vi "Drivetrain Loop.vi"   [LabVIEW 2016]
uses:
  <vilib>/Rock Robotics/WPI/ThirdParty/Sensors/navX/_TypeDefs/FRIC_navX_DeviceNumbersTypeDef.ctl
  Common Code/PID Gains.ctl
  Common Code/Utilities/Change Detect Int.vi
  Common Code/Utilities/Change Detect Boolean.vi
  Robot Global Data.vi
  <vilib>/Rock Robotics/WPI/Solenoid/Deprecated/WPI_SolenoidSetBool.vi
types:
  T1 = typedef "FRIC_navX_DeviceNumbersTypeDef.ctl" = enum16{"Dev0", "Dev1", "Dev2", "Dev3"}
  T2 = typedef "Drivetrain Command Cluster.ctl" = cluster{"Drivetrain Mode":T3, "Heading Target":dbl, "Turn Power":dbl, "Y Power":dbl, "Center Piston Down?":bool, "Traction?":bool, "Strafe Power":dbl, "Zero Gyro":bool, "Distance Target":dbl, "Strafe Correct":bool, "Y Max Output":dbl, "Y Min Output":dbl, "X Max Output":dbl, "X Min Output":dbl, "Z Max Output":dbl, "Z Min Output":dbl, "Z Target":dbl, "Brake?":bool}
  T3 = typedef "Drivetrain Mode.ctl" = enum16{"Manual", "Gyro Steer", "Distance Drive", "Translate Drive", "Goal Vision Align", "PID Drive"}
  T4 = typedef "Dashboard Control Data.ctl" = cluster{"Drivetrain Settings":T5, "Intake Presets ":T8, "Shooter Presets":T9, "Vision Target Packet":T10, "Auton Presets":cluster{"Start Position":dbl}, "Drivetrain Encoder Values":T11, "Drivetrain Encoder Settings":cluster{"Left Tick Constant":dbl, "Right Tick Contant":dbl, "Reset Encoders":bool, "Center Tick Constant":dbl}, "Zero Gyro":bool, "Vision Timeout":dbl, "Pressure M":dbl, "Pressure B":dbl, "Auto Agitator":T13, "Climber Settings":T14, "LEDs":T15}
  T5 = typedef "Drivetrain Settings.ctl" = cluster{"Gyro Tolerance":dbl, "Gyro Steer PID Gains":T6, "Y Power Multiplier":dbl, "Turn Power Multiplier":dbl, "Gyro Output":dbl, "Creep Rate":dbl, "Distance Drive PID Gains":T6, "Distance Tolerance":dbl, "Distance Output":dbl, "Strafe Threshold":dbl, "Strafe Correct":bool, "Strafe Corect Tolerance":dbl, "Translate Drive PID Gains":T6, "Strafe Output":dbl, "SC Right":dbl, "SC Left":dbl, "Use Gyro":bool, "Constant Power":bool, "Strafe Power":dbl, "Input Modifier":T7}
  T6 = typedef "PID Gains.ctl" = cluster{"proportional gain (Kc)":dbl, "integral time (Ti, min)":dbl, "derivative time (Td, min)":dbl}
  T7 = typedef "Input Modifier.ctl" = enum16{"None", "Square", "Cube"}
  T8 = typedef "Intake Presets.ctl" = cluster{"Intake Speed ":dbl, "Outake Speed":dbl, "Current Trip Delay":dbl, "Max Current":dbl, "Gear Outtake Motor Delay":dbl, "Gear Intake Motor Delay":dbl, "Gear Intake?":bool, "Gear Intake Pull Up Speed":dbl}
  T9 = typedef "Shooter Presets.ctl" = cluster{"Key Shot":cluster{"RPM ":dbl, "Hood?":bool}, "Distance Shot":cluster{"RPM":dbl, "Hood?":bool}, "RPM Tolerance":dbl, "Unstuck Delay Time ":dbl, "Initial RPM Increase":dbl, "Warmup Delay":dbl, "Faster Time":dbl, "Shooter PID Gains":cluster{"P":dbl, "I":dbl, "D":dbl, "FF":dbl, "Ramp Rate":dbl, "I Zone":dbl}, "Unstuck Trigger Power":dbl, "Trigger Power":dbl, "Unstuck RPM":dbl, "Agitator Active Power":dbl, "Agitator Idle Power":dbl}
  T10 = typedef "Vision Target Packet.ctl" = cluster{"Robot Center":dbl, "Center X":dbl, "Center Y":dbl, "Angle":dbl, "Distance":dbl, "Found Target?":bool}
  T11 = typedef "Drivetrain Encoder Values.ctl" = cluster{"Left Encoder":T12, "Center Encoder":T12, "Right Encoder":T12}
  T12 = typedef "Encoder Values.ctl" = cluster{"Distance":dbl, "Speed":dbl, "Tick":dbl}
  T13 = typedef "Auto Agitator Settings.ctl" = cluster{"Enable Auto Agitation":bool, "Continuous Stir":bool, "Continuous Intake":bool, "Alternate In/Outtake":bool, "Wing Delay":dbl, "Stir Delay":dbl, "Intake Delay":dbl, "Wing On Time":dbl, "Wing Off Time":dbl, "Stir On Time":dbl, "Stir Off Time":dbl, "Intake On Time":dbl, "Intake Off Time":dbl, "Stir Power":dbl, "Intake Power":dbl, "Outtake Power":dbl, "Intake Run Time":dbl, "Outtake Run Time":dbl, "Wing$":bool, "Intake":bool, "Stirrer":bool}
  T14 = typedef "Climber Settings.ctl" = cluster{"Climber Power":dbl, "Max Current":dbl, "Avoid Current Trip?":bool}
  T15 = typedef "LED Global Data.ctl" = cluster{"Back":cluster{"Default":string, "Traction":string, "Gear Ready":string, "Break On":string, "Gear Loaded":string}, "Front":cluster{"Default":string, "Traction":string, "Gear Ready":string, "Break On":string, "Gear Loaded":string}}
  T16 = typedef "Goal Vision Packet.ctl" = cluster{"Distance":dbl, "Angle":dbl, "Found Target?":bool}
  T17 = cluster{"Yaw":dbl, "Roll":dbl, "Pitch":dbl, "Heading":dbl, "Fused Heading":dbl}
  T18 = cluster{"Target Heading":dbl, "Target Distance":dbl, "Target Translation":dbl}
  T19 = cluster{"Gyro PID Gains":T6, "Distance PID Gains":T6, "Strafe PID Gains":T6}
  T20 = cluster{"Y Max":dbl, "X Max":dbl, "Z Max":dbl, "Y Min":dbl, "X Min":dbl, "Z Min":dbl}
  T21 = cluster{"Distance Tolerance":dbl, "Strafe Tolerance":dbl, "Gyro Tolerance":dbl}
  T22 = typedef "WPI_SolenoidDevRef.ctl" = cluster{"DevStatus":errorcluster, "Pneumatics Control Module":u8, "Forward Solenoid Channel":T23, "Reverse Solenoid Channel":T23}
  T23 = typedef "WPI_SolenoidChannel.ctl" = enum8{"Solenoid 0", "Solenoid 1", "Solenoid 2", "Solenoid 3", "Solenoid 4", "Solenoid 5", "Solenoid 6", "Solenoid 7", "Invalid"}
  T24 = typedef "WPI_MotorControlDeviceRef.ctl" = cluster{"DeviceStatus":errorcluster, "Type":T25, "PWM":cluster{"PWM Channel":T26, "DeadBand":T27}, "CAN":cluster{"Device Number":u8, "SetOutput VI Ref":variant, "GetOutput VI Ref":variant, "Enable VI Ref":variant, "Disable VI Ref":variant, "Data":variant}, "Invert":bool}
  T25 = typedef "WPI_MotorControlType.ctl" = enum16{"PWM", "CAN"}
  T26 = typedef "FPGA_DIOPWMChannel.ctl" = enum8{"PWM 0", "PWM 1", "PWM 2", "PWM 3", "PWM 4", "PWM 5", "PWM 6", "PWM 7", "PWM 8", "PWM 9", "PWM MXP 0", "PWM MXP 1", "PWM MXP 2", "PWM MXP 3", "PWM MXP 4", "PWM MXP 5", "PWM MXP 6", "PWM MXP 7", "PWM MXP 8", "PWM MXP 9", "Invalid"}
  T27 = typedef "WPI_PWMDeadband.ctl" = cluster{"Name":string, "maxPositivePwm":i32, "minPositivePwm":i32, "centerPwm":i32, "maxNegativePwm":i32, "minNegativePwm":i32, "angularRange":u16}
  T28 = typedef "Drivetrain Status Cluster.ctl" = cluster{"Drivetrain Mode":enum16{"Manual", "Gyro Steer"}, "Y (Throttle)":dbl, "X (Steer)":dbl, "Z (Strafe)":dbl, "Heading Target":dbl, "Center Piston Down?":bool, "Traction?":bool, "Gyro Steer Finished?":bool, "Distance Drive Finished?":bool, "Gyro":dbl, "Distance Target":dbl, "Y Max Output":dbl, "Y Min Output":dbl, "X Max Output":dbl, "X Min Output":dbl, "Z Max Output":dbl, "Z Min Output":dbl, "Translation Target":dbl, "Translation Drive Finished?":bool, "PID Auto Drive Finished?":bool, "Brake?":bool, "Vision Aligned?":bool, "Creep Mode Engaged?":bool}
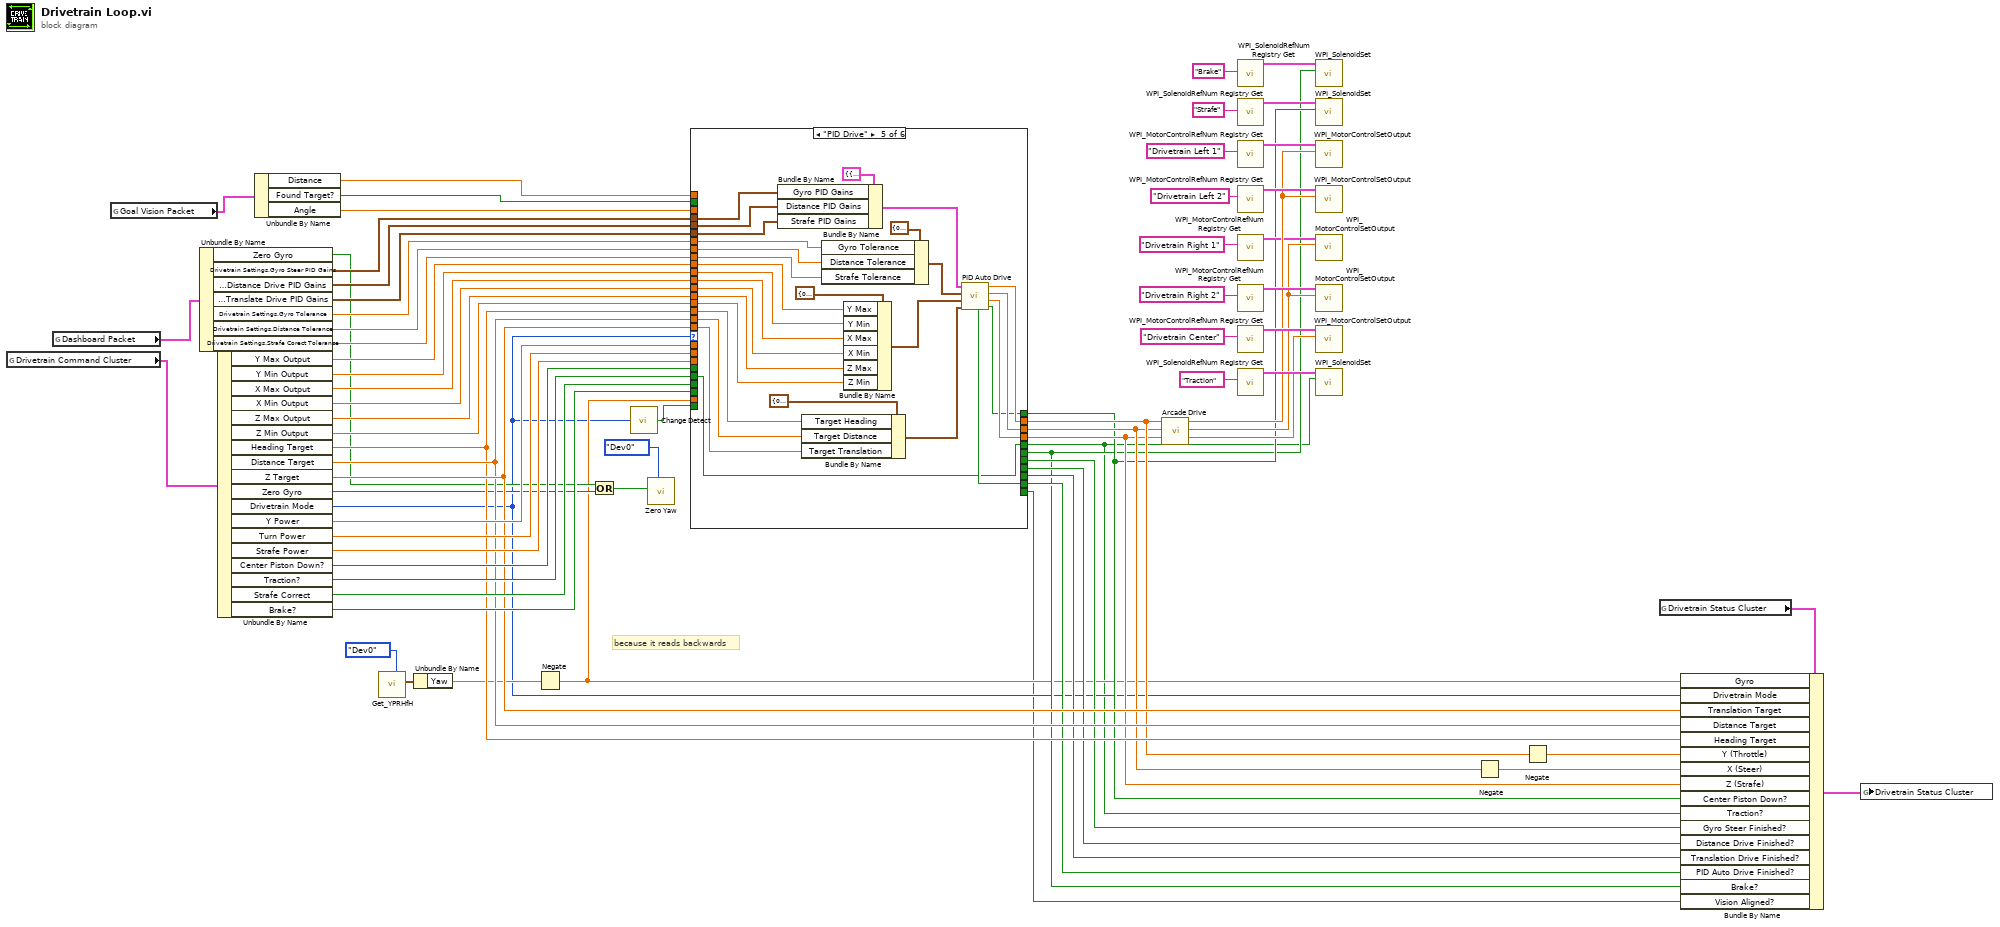
[diagram p0: block diagram]
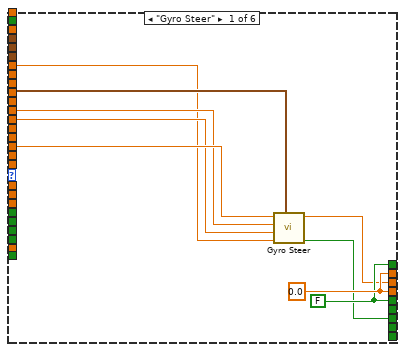
[diagram p2: hidden frame]
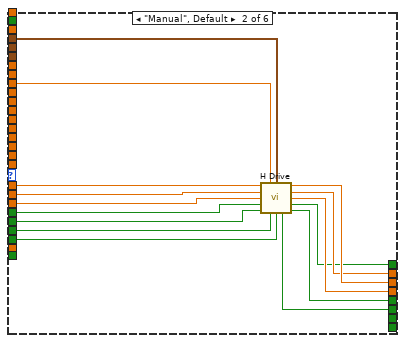
[diagram p3: hidden frame]
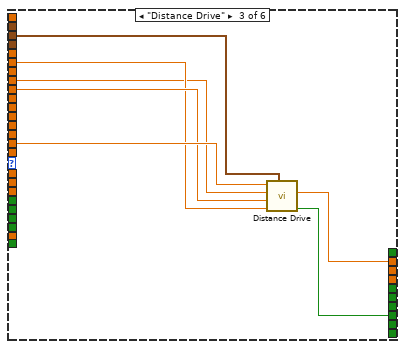
[diagram p4: hidden frame]
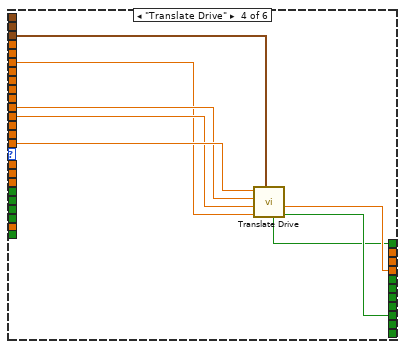
[diagram p5: hidden frame]
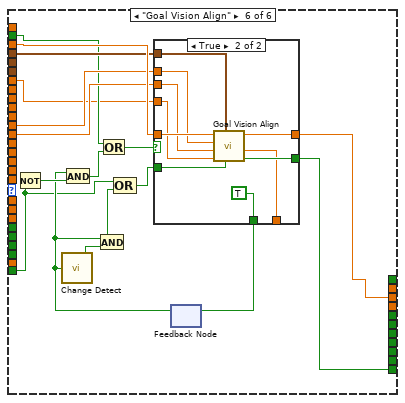
[diagram p6: hidden frame]
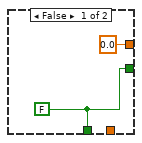
[diagram p7: hidden frame]
diagram:
  # "because it reads backwards"
  n1 = global read "Robot Global Data.vi" "Drivetrain Command Cluster"() -> (w67:T2)
  n2 = global read "Robot Global Data.vi" "Dashboard Packet"() -> (w55:T4)
  n3 = global read "Robot Global Data.vi" "Goal Vision Packet"() -> (w10:T16)
  n4 = Unbundle By Name(w55) -> ("Zero Gyro"=w16:bool, "Drivetrain Settings.Gyro Steer PID Gains"=w54:T6, "Drivetrain Settings.Distance Drive PID Gains"=w53:T6, "Drivetrain Settings.Translate Drive PID Gains"=w42:T6, "Drivetrain Settings.Gyro Tolerance"=w52:dbl, "Drivetrain Settings.Distance Tolerance"=w51:dbl, "Drivetrain Settings.Strafe Corect Tolerance"=w50:dbl)
  n5 = Unbundle By Name(w67) -> ("Y Max Output"=w48:dbl, "Y Min Output"=w47:dbl, "X Max Output"=w45:dbl, "X Min Output"=w46:dbl, "Z Max Output"=w44:dbl, "Z Min Output"=w43:dbl, "Heading Target"=w28:dbl, "Distance Target"=w29:dbl, "Z Target"=w30:dbl, "Zero Gyro"=w17:bool, "Drivetrain Mode"=w4:T3, "Y Power"=w58:dbl, "Turn Power"=w57:dbl, "Strafe Power"=w56:dbl, "Center Piston Down?"=w60:bool, "Traction?"=w59:bool, "Strafe Correct"=w49:bool, "Brake?"=w33:bool)
  n6 = Unbundle By Name(w10) -> ("Distance"=w6:dbl, "Found Target?"=w5:bool, "Angle"=w9:dbl)
  n7 = call <vilib>:"Get_YPRHfH.vi"("Device Number"=FRIC_navX_DeviceNumbersTypeDef."Dev0") -> ("YRPHfH"=w20:T17)  [unwired: 10 in]
  n8 = Unbundle By Name(w20) -> ("Yaw"=w8:dbl)
  n9 = Negate(x=w8) -> (-x=w7:dbl)
  n10 = Or(x=w16, y=w17) -> (x .or. y?=w15:bool)
  n11 = call-poly "Change Detect.vi"("In"=w4) -> ("Changed?"=w3:bool)
  n12 = call <vilib>:"Zero Yaw.vi"("Device Number"=FRIC_navX_DeviceNumbersTypeDef."Dev0", "Zero"=w15) -> ()  [unwired: 10 in]
  n13 = case shown="\"PID Drive\"" w4 {
    tunnel: [w80 w86 w102 _ w115 _] -> w27
    tunnel: [w78 w87 _ _ w114 w140] -> w26
    tunnel: [w80 w85 _ w105 w116 _] -> w25
    tunnel: [w79 w83 _ w103 w113 _] -> w24
    tunnel: [w79 w84 _ _ w111 _] -> w1
    tunnel: w58 -> [_ w95 _ _ _ _]
    tunnel: w57 -> [_ w94 _ _ _ _]
    tunnel: w56 -> [_ w93 _ _ _ _]
    tunnel: w60 -> [_ w92 _ _ _ _]
    tunnel: w59 -> [_ w91 _ _ w111 _]
    tunnel: w54 -> [w76 w90 _ _ w135 w149]
    tunnel: w53 -> [_ _ w100 _ w134 _]
    tunnel: w52 -> [w72 _ _ _ w128 w145]
    tunnel: w51 -> [_ _ w97 _ w127 _]
    tunnel: w28 -> [w75 _ _ _ w119 _]
    tunnel: w29 -> [_ _ w99 _ w118 _]
    tunnel: [w77 _ _ _ _ _] -> w23
    tunnel: [_ _ w101 _ _ _] -> w22
    tunnel: w50 -> [_ w89 _ w106 w126 _]
    tunnel: w49 -> [_ w88 _ _ _ _]
    tunnel: w48 -> [_ _ w96 _ w125 _]
    tunnel: w47 -> [_ _ w98 _ w124 _]
    tunnel: w45 -> [w74 _ _ _ w123 w148]
    tunnel: w46 -> [w73 _ _ _ w122 w147]
    tunnel: w44 -> [_ _ _ w108 w121 _]
    tunnel: w43 -> [_ _ _ w107 w120 _]
    tunnel: w42 -> [_ _ _ w110 w133 _]
    tunnel: w30 -> [_ _ _ w109 w117 _]
    tunnel: [_ _ _ w104 _ _] -> w21
    tunnel: w33 -> [_ w82 _ _ _ _]
    tunnel: [_ w81 _ _ _ _] -> w11
    tunnel: [_ _ _ _ w112 _] -> w12
    tunnel: w9 -> [_ _ _ _ _ w156]
    tunnel: w7 -> [_ _ _ _ _ _]
    tunnel: w6 -> [_ _ _ _ _ _]
    tunnel: w5 -> [_ _ _ _ _ w146]
    tunnel: w3 -> [_ _ _ _ _ w143]
    tunnel: [_ _ _ _ _ w141] -> w2
    frame "Gyro Steer" {
      w80 = 0.0 ("Center Motor Output")
      w79 = FALSE ("HDrive Piston")
      n14 = call "Gyro Steer.vi"("PID gains"=w76, "Gyro Tolerance"=w72, "X Min Output"=w73, "X Max Output"=w74, "Target Heading"=w75) -> ("Finished?"=w77:bool, "X out"=w78:dbl)  [unwired: 5 in]
    }
    frame "Manual", Default {
      n15 = call "H Drive.vi"("Y Power"=w95, "Strafe Correct Tolerance"=w89, "Strafe Correct PID Gains"=w90, "Turn Power"=w94, "Strafe Power"=w93, "Center Piston Down?"=w92, "Traction?"=w91, "Strafe Correct"=w88, "Brake?"=w82) -> ("X Out"=w87:dbl, "Y out"=w86:dbl, "Center Motor Output"=w85:dbl, "HDrive Piston"=w83:bool, "Brake."=w81:bool, "Grasshopper Pistons"=w84:bool)  [unwired: 1 in]
    }
    frame "Distance Drive" {
      n16 = call "Distance Drive.vi"("PID gains"=w100, "Distance Tolerance"=w97, "Y Min Output"=w98, "Y Max Output"=w96, "Distance Target"=w99) -> ("Finished?"=w101:bool, "Y Output"=w102:dbl)  [unwired: 5 in]
    }
    frame "Translate Drive" {
      n17 = call "Translate Drive.vi"("Translation PID Gains"=w110, "Translation Tolerance"=w106, "Z Min Output"=w107, "Z Max Output"=w108, "Target Translation"=w109) -> ("Finished?"=w104:bool, "Z Out"=w105:dbl, "Center Piston Down?"=w103:bool)  [unwired: 4 in]
    }
    frame "PID Drive" {
      n18 = Bundle By Name(cluster=T19 {"Gyro PID Gains"={"proportional gain (Kc)"=1.0, "integral time (Ti, min)"=0.01, "derivative time (Td, min)"=0.0}, "Distance PID Gains"={"proportional gain (Kc)"=1.0, "integral time (Ti, min)"=0.01, "derivative time (Td, min)"=0.0}, "Strafe PID Gains"={"proportional gain (Kc)"=1.0, "integral time (Ti, min)"=0.01, "derivative time (Td, min)"=0.0}} ("PID Gains"), "Gyro PID Gains"=w135, "Distance PID Gains"=w134, "Strafe PID Gains"=w133) -> (w136:T19)
      n19 = Bundle By Name(cluster=T18 {"Target Heading"=0.0, "Target Distance"=0.0, "Target Translation"=0.0} ("Targets"), "Target Heading"=w119, "Target Distance"=w118, "Target Translation"=w117) -> (w129:T18)
      n20 = Bundle By Name(cluster=T21 {"Distance Tolerance"=0.0, "Strafe Tolerance"=0.0, "Gyro Tolerance"=0.0} ("Tolerances"), "Gyro Tolerance"=w128, "Distance Tolerance"=w127, "Strafe Tolerance"=w126) -> (w132:T21)
      n21 = Bundle By Name(cluster=T20 {"Y Max"=0.0, "X Max"=0.0, "Z Max"=0.0, "Y Min"=0.0, "X Min"=0.0, "Z Min"=0.0} ("Motor Values"), "Y Max"=w125, "Y Min"=w124, "X Max"=w123, "X Min"=w122, "Z Max"=w121, "Z Min"=w120) -> (w131:T20)
      n22 = call "PID Auto Drive.vi"("Targets"=w129, "Motor Values"=w131, "Tolerances"=w132, "PID Gains"=w136) -> ("Center Piston Down?"=w113:bool, "Z Out"=w116:dbl, "X Out"=w114:dbl, "Y Out"=w115:dbl, "Finished?"=w112:bool)  [unwired: 3 in]
    }
    frame "Goal Vision Align" {
      n23 = Not(x=w143) -> (.not. x?=w153:bool)
      n24 = feedback #1() -> (w152:bool)  [unwired: 1 in]
      n25 = call-poly "Change Detect.vi"("In"=w152) -> ("Changed?"=w154:bool)
      n26 = And(x=w152, y=w153) -> (x .and. y?=w151:bool)
      n27 = And(x=w152, y=w154) -> (x .and. y?=w144:bool)
      n28 = Or(x=w146, y=w151) -> (x .or. y?=w155:bool)
      n29 = Compound Arithmetic op=OR(w143, w144) -> (w142:bool)
      n30 = case shown="True" w155 {
        tunnel: w156 -> [_ w168]
        tunnel: [0.0 ("X Out") w167] -> w140
        tunnel: [w157 w166] -> w141
        tunnel: w142 -> [_ w160]
        tunnel: [w157 TRUE] -> w150
        tunnel: [_ w164] -> _
        tunnel: w149 -> [_ w163]
        tunnel: w148 -> [_ w162]
        tunnel: w147 -> [_ w161]
        tunnel: w145 -> [_ w159]
        frame False {
          w157 = FALSE
        }
        frame True {
          n31 = call "Goal Vision Align.vi"("Reinitialize?"=w160, "PID gains"=w163, "Gyro Tolerance"=w159, "X Min"=w161, "X Max"=w162, "Goal Angle Difference"=w168) -> ("Finished?"=w166:bool, "Heading Target"=w164:dbl, "X Out"=w167:dbl)  [unwired: 3 in]
        }
      }
      n32 = feedback-in #1(w150) -> ()
    }
  }
  n33 = call "Arcade Drive.vi"("Turn Power"=w26, "Y Power"=w27) -> ("Right Motor Output"=w36:dbl, "Left Motor Output"=w40:dbl)  [unwired: 8 in]
  n34 = call <vilib>:"WPI_SolenoidRefNum Registry Get.vi"("refnum name"="Brake") -> ("SolenoidDevRef"=w34:T22)  [unwired: 9 in, 1 out]
  n35 = call <vilib>:"WPI_SolenoidRefNum Registry Get.vi"("refnum name"="Strafe") -> ("SolenoidDevRef"=w64:T22)  [unwired: 9 in, 1 out]
  n36 = call <vilib>:"WPI_MotorControlRefNum Registry Get.vi"("refnum name"="Drivetrain Left 1") -> ("MotorControlDevRef"=w71:T24)  [unwired: 9 in, 1 out]
  n37 = call <vilib>:"WPI_MotorControlRefNum Registry Get.vi"("refnum name"="Drivetrain Left 2") -> ("MotorControlDevRef"=w41:T24)  [unwired: 9 in, 1 out]
  n38 = call <vilib>:"WPI_MotorControlRefNum Registry Get.vi"("refnum name"="Drivetrain Right 1") -> ("MotorControlDevRef"=w37:T24)  [unwired: 9 in, 1 out]
  n39 = call <vilib>:"WPI_MotorControlRefNum Registry Get.vi"("refnum name"="Drivetrain Right 2") -> ("MotorControlDevRef"=w70:T24)  [unwired: 9 in, 1 out]
  n40 = call <vilib>:"WPI_MotorControlRefNum Registry Get.vi"("refnum name"="Drivetrain Center") -> ("MotorControlDevRef"=w65:T24)  [unwired: 9 in, 1 out]
  n41 = call <vilib>:"WPI_SolenoidRefNum Registry Get.vi"("refnum name"="Traction") -> ("SolenoidDevRef"=w63:T22)  [unwired: 9 in, 1 out]
  n42 = call-poly <vilib>:"WPI_SolenoidSet.vi"("Value"=w11, "SolenoidDevRef"=w34) -> ()  [unwired: 8 in, 2 out]
  n43 = call-poly <vilib>:"WPI_SolenoidSet.vi"("Value"=w24, "SolenoidDevRef"=w64) -> ()  [unwired: 8 in, 2 out]
  n44 = call <vilib>:"WPI_MotorControlSetOutput.vi"("Output"=w40, "MotorControlDevRef"=w71) -> ()  [unwired: 7 in, 3 out]
  n45 = call <vilib>:"WPI_MotorControlSetOutput.vi"("Output"=w40, "MotorControlDevRef"=w41) -> ()  [unwired: 7 in, 3 out]
  n46 = call <vilib>:"WPI_MotorControlSetOutput.vi"("Output"=w36, "MotorControlDevRef"=w37) -> ()  [unwired: 7 in, 3 out]
  n47 = call <vilib>:"WPI_MotorControlSetOutput.vi"("Output"=w36, "MotorControlDevRef"=w70) -> ()  [unwired: 7 in, 3 out]
  n48 = call <vilib>:"WPI_MotorControlSetOutput.vi"("Output"=w25, "MotorControlDevRef"=w65) -> ()  [unwired: 7 in, 3 out]
  n49 = call-poly <vilib>:"WPI_SolenoidSet.vi"("Value"=w1, "SolenoidDevRef"=w63) -> ()  [unwired: 8 in, 2 out]
  n50 = Negate(x=w26) -> (-x=w18:dbl)
  n51 = Negate(x=w27) -> (-x=w19:dbl)
  n52 = global read "Robot Global Data.vi" "Drivetrain Status Cluster"() -> (w32:T28)
  n53 = Bundle By Name(cluster=w32, "Gyro"=w7, "Drivetrain Mode"=w4, "Translation Target"=w30, "Distance Target"=w29, "Heading Target"=w28, "Y (Throttle)"=w19, "X (Steer)"=w18, "Z (Strafe)"=w25, "Center Piston Down?"=w24, "Traction?"=w1, "Gyro Steer Finished?"=w23, "Distance Drive Finished?"=w22, "Translation Drive Finished?"=w21, "PID Auto Drive Finished?"=w12, "Brake?"=w11, "Vision Aligned?"=w2) -> (w31:T28)
  n54 = global write "Robot Global Data.vi" "Drivetrain Status Cluster"(w31) -> ()
